vi "Init.vi"(7 "EDS":refnum<class "Electronic Datasheet.lvclass">, 8 "error in":errorcluster, 10 "OD Entry":refnum<class "OD Entry.lvclass">, 11 "PDO Mapping in":refnum<class "PDO Mapping.lvclass">) -> (0 "error out":errorcluster, 3 "PDO Mapping out":refnum<class "PDO Mapping.lvclass">)   [LabVIEW 2019, in "PDO Grid.lvlib" / "PDO Mapping.lvclass"]
uses:
  PDO Mapping.lvclass
  Core/OD Entry/OD Entry.lvclass
  Electronic Datasheet/Electronic Datasheet.lvclass
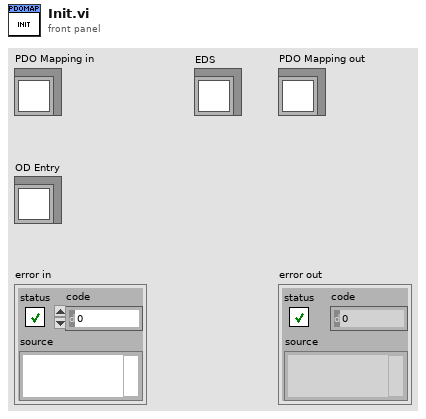
[diagram p1: front panel]
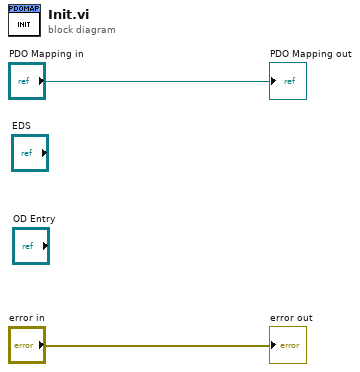
[diagram p0: block diagram]
diagram:
  "error out" <- "error in"
  "PDO Mapping out" <- "PDO Mapping in"
